vi "process.vi"(8 "error in (no error)":errorcluster, 10 "input":sgl[][](array[numeric]), 11 "DL090628DSSTraceProcessor in":refnum<class "TraceProcessorDL090628DSS.lvclass">) -> (0 "error out":errorcluster, 2 "traces":sgl[][](graph), 3 "DL090628DSSTraceProcessor out":refnum<class "TraceProcessorDL090628DSS.lvclass">)   [LabVIEW 2010, in "TraceProcessorDL090628DSS.lvclass"]
uses:
  TraceProcessorDL090628DSS.lvclass
  TraceProcessorDL090628DSS.lvclass/TraceProcessorDL090628DSS.ctl
  <vilib>/Analysis/NI_AALBase.lvlib
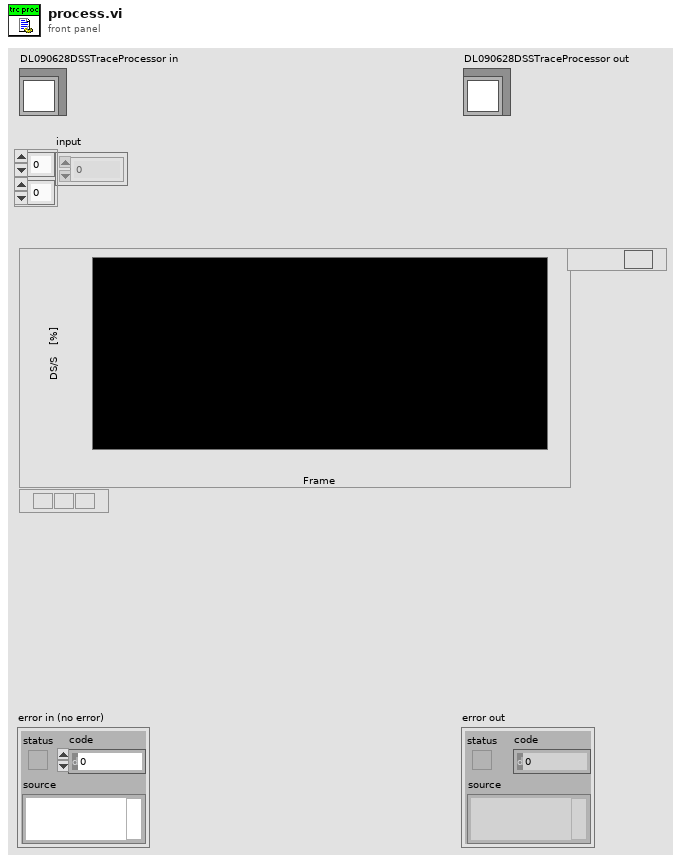
[diagram p1: front panel]
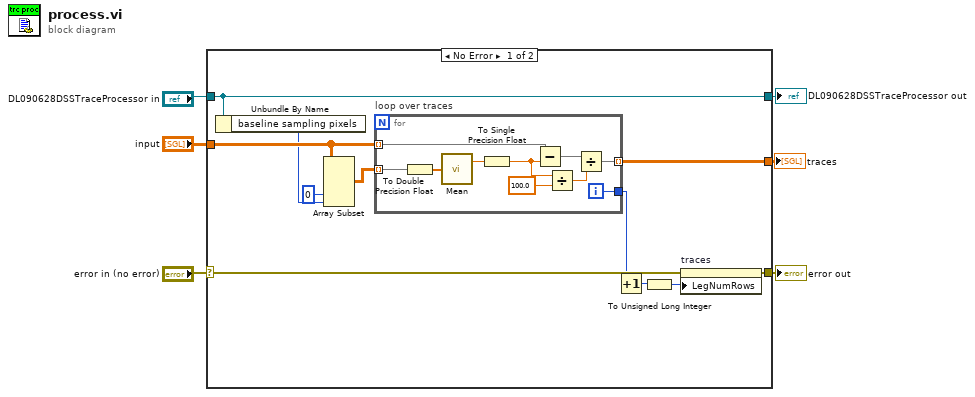
[diagram p0: block diagram]
diagram:
  n1 = case shown="No Error" "error in (no error)" {
    selector: "error in (no error)" -> [w11 w29]
    tunnel: [w10 w29] -> w5
    tunnel: [w17 w30] -> w3
    tunnel: "DL090628DSSTraceProcessor in" -> [w17 w30]
    tunnel: "input" -> [w15 w28]
    tunnel: [w16 w28] -> w1
    frame No Error {
      n2 = Unbundle By Name(w17) -> ("baseline sampling pixels"=w14:i32)
      n3 = Array Subset(array=w15, index (col)=0 ("index"), length (col)=w14) -> (w12:sgl[][])  [unwired: 2 in]
      n4 = for "loop over traces" {
        tunnel: w12 -> [w23] mode=indexing
        tunnel: [w24] -> w16 mode=indexing
        tunnel: w15 -> [w26] mode=indexing
        tunnel: [w18] -> w9
        i -> [w18]
        n5 = To Double Precision Float(number=w23) -> (double precision float=w22:dbl[])
        n6 = call <vilib>:"Mean.vi"("X"=w22) -> ("mean"=w25:dbl)  [unwired: 1 out]
        n7 = To Single Precision Float(number=w25) -> (single precision float=w21:sgl)
        n8 = Subtract(x=w26, y=w21) -> (x-y=w27:sgl[])
        n9 = Divide(x=w21, y=sgl 100.0) -> (x/y=w19:sgl)
        n10 = Divide(x=w27, y=w19) -> (x/y=w24:sgl[])
      }
      n11 = Increment(x=w9) -> (x+1=w8:i32)
      n12 = To Unsigned Long Integer(number=w8) -> (unsigned 32bit integer=w7:u32)
      n13 = property on="traces" class="WFGraph (strict)"(error in=w11, "LegNumRows"=w7) -> (error out=w10:errorcluster)  [unwired: 1 in, 1 out]
    }
    frame Error {
    }
  }
  "error out" <- w5
  "DL090628DSSTraceProcessor out" <- w3
  "traces" <- w1
